vi "jiga.vi"() -> ()   [LabVIEW 2014]
uses:
  stateCtl.ctl
  <vilib>/Instr/_visa.llb/VISA Configure Serial Port (Instr).vi
panel:
  in  "Digital\nOutput 3":bool
  out "Led3":bool
  out "ASCII Read":string
  in  "Filter\nRead":bool
  out "Led0":bool
  out "ASCII Digital":string
  out "ASCII Analog 2":string
  out "ASCII Analog 1":string
  in  "AnalogOutput 2 \n      DutyCycle":dbl(slide) scale=0.0..100.0
  out "S7":dbl
  in  "AnalogOutput 1 \n      DutyCycle":dbl(slide) scale=0.0..100.0
  out "Led2":bool
  in  "Digital\nOutput 2":bool
  out "Led1":bool
  in  "Digital\nOutput 1":bool
  out "S6":dbl
  out "S5":dbl
  out "S4":dbl
  out "S3":dbl
  out "S2":dbl
  out "S1":dbl
  out "S0":dbl
  in  "Tab Control":T1(tab)
  out "Frequency":dbl(graph)
  out "Temperature 1":dbl(graph)
  out "Temperature 2":dbl(graph)
  out "Load Cell 1":dbl(graph)
  out "Load Cell 2":dbl(graph)
  out "Vibration":dbl(graph)
  out "Analog Output 1":dbl(graph)
  out "Analog Output 2":dbl(graph)
  out "exitLed":bool
  out "statusBar":string="     "
  in  "startButton":bool
  out "stopLed":bool
  out "startLed":bool
  in  "VISA Serial Port":refnum<visa-resource-name>
  in  "exitButton":bool
  in  "stopButton":bool
  out "FE":string
  out "FP":string
  out "isRunning":bool
  out "state":T2=enum."exit"
  # "`"
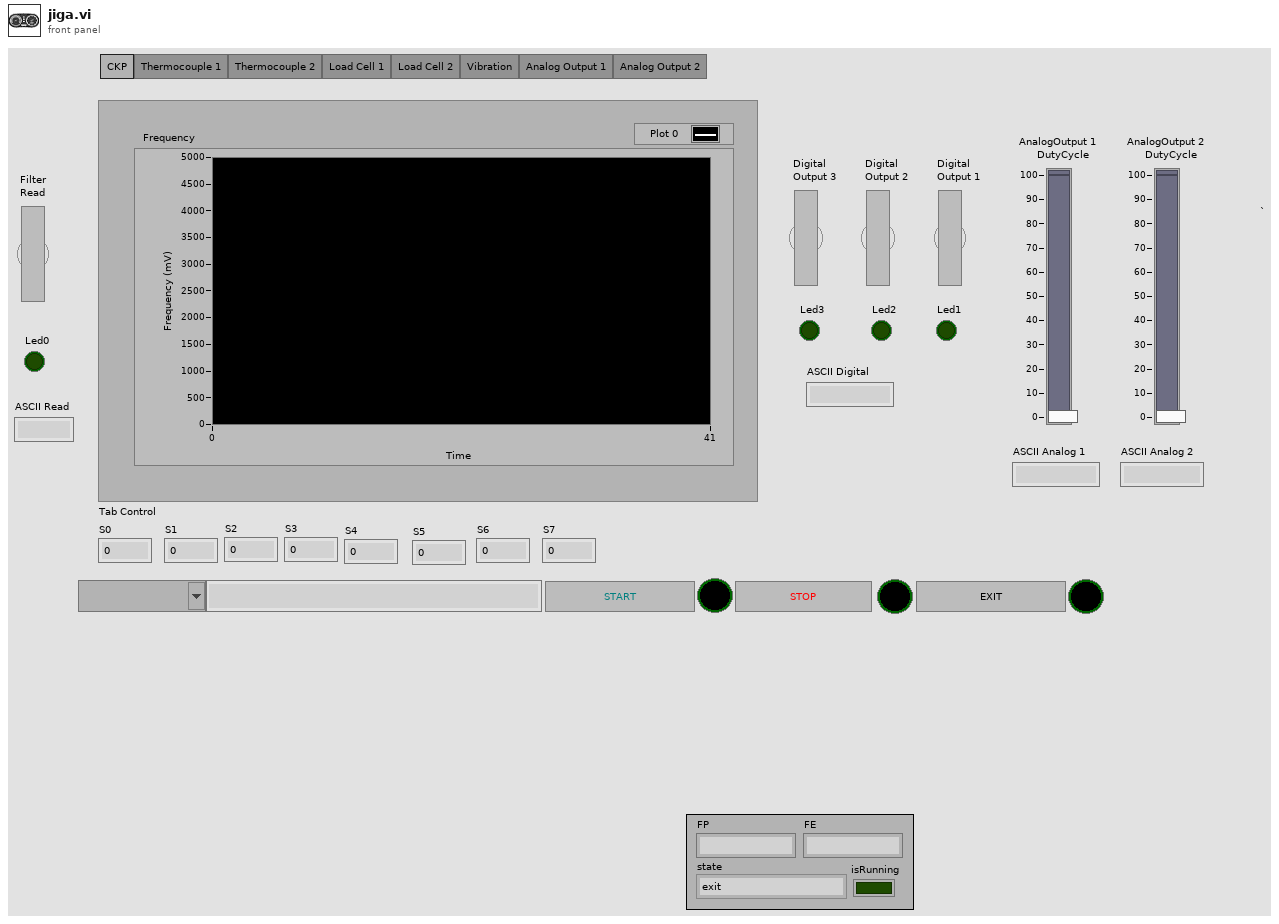
[diagram p1: front panel]
types:
  T1 = enum32{"CKP", "Thermocouple 1", "Thermocouple 2", "Load Cell 1", "Load Cell 2", "Vibration", "Analog Output 1", "Analog Output 2"}
  T2 = typedef "stateCtl.ctl" = enum16{"init", "ready", "running", "stopped", "exit"}
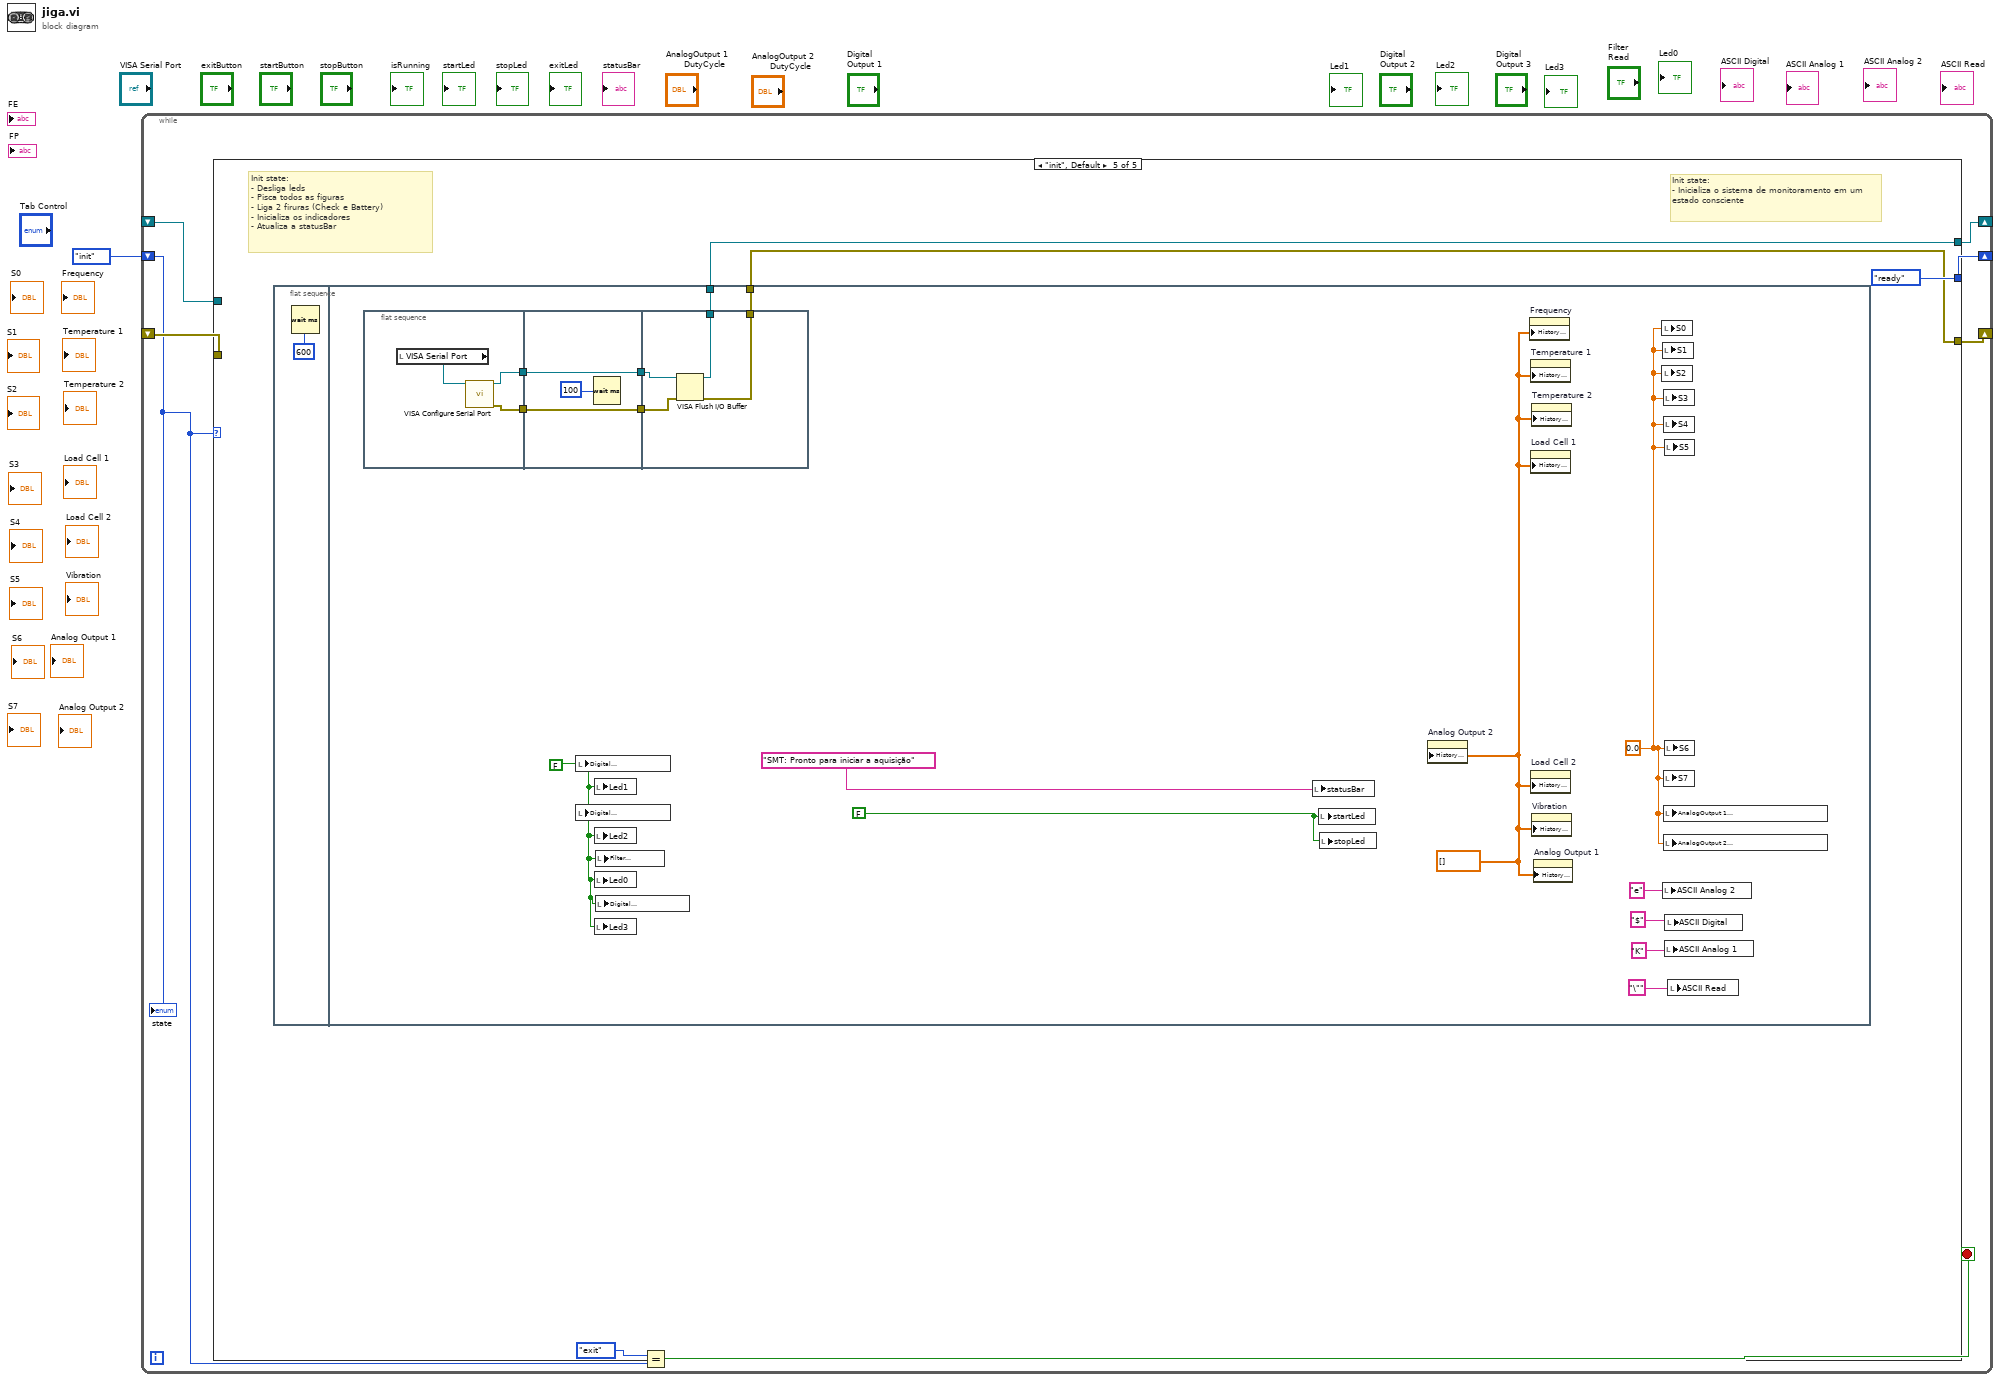
[diagram p0: block diagram]
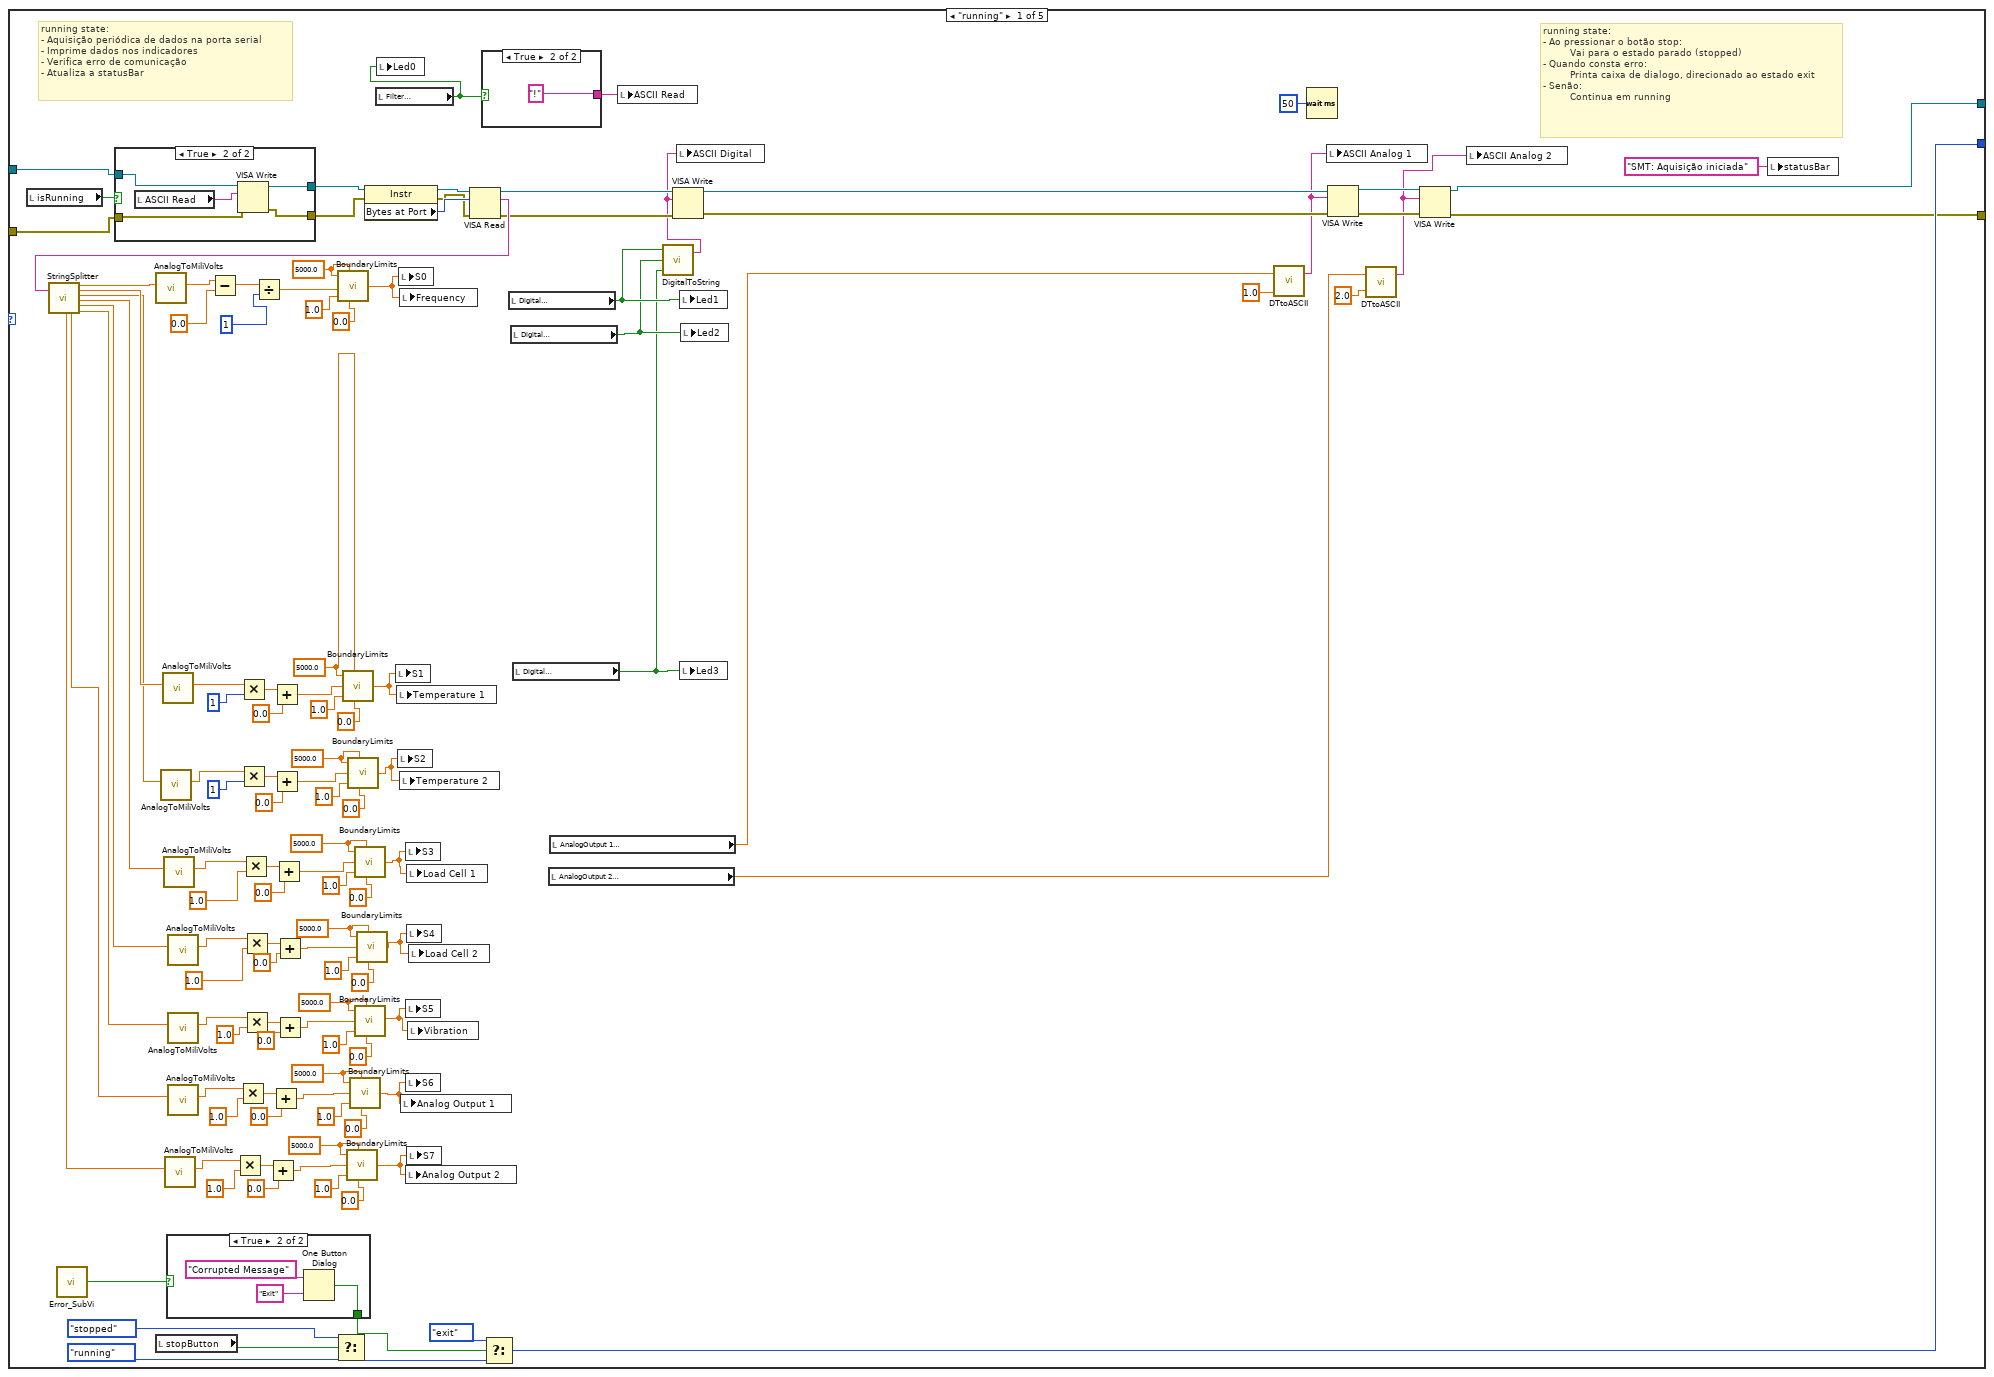
[diagram p2: hidden frame]
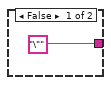
[diagram p3: hidden frame]
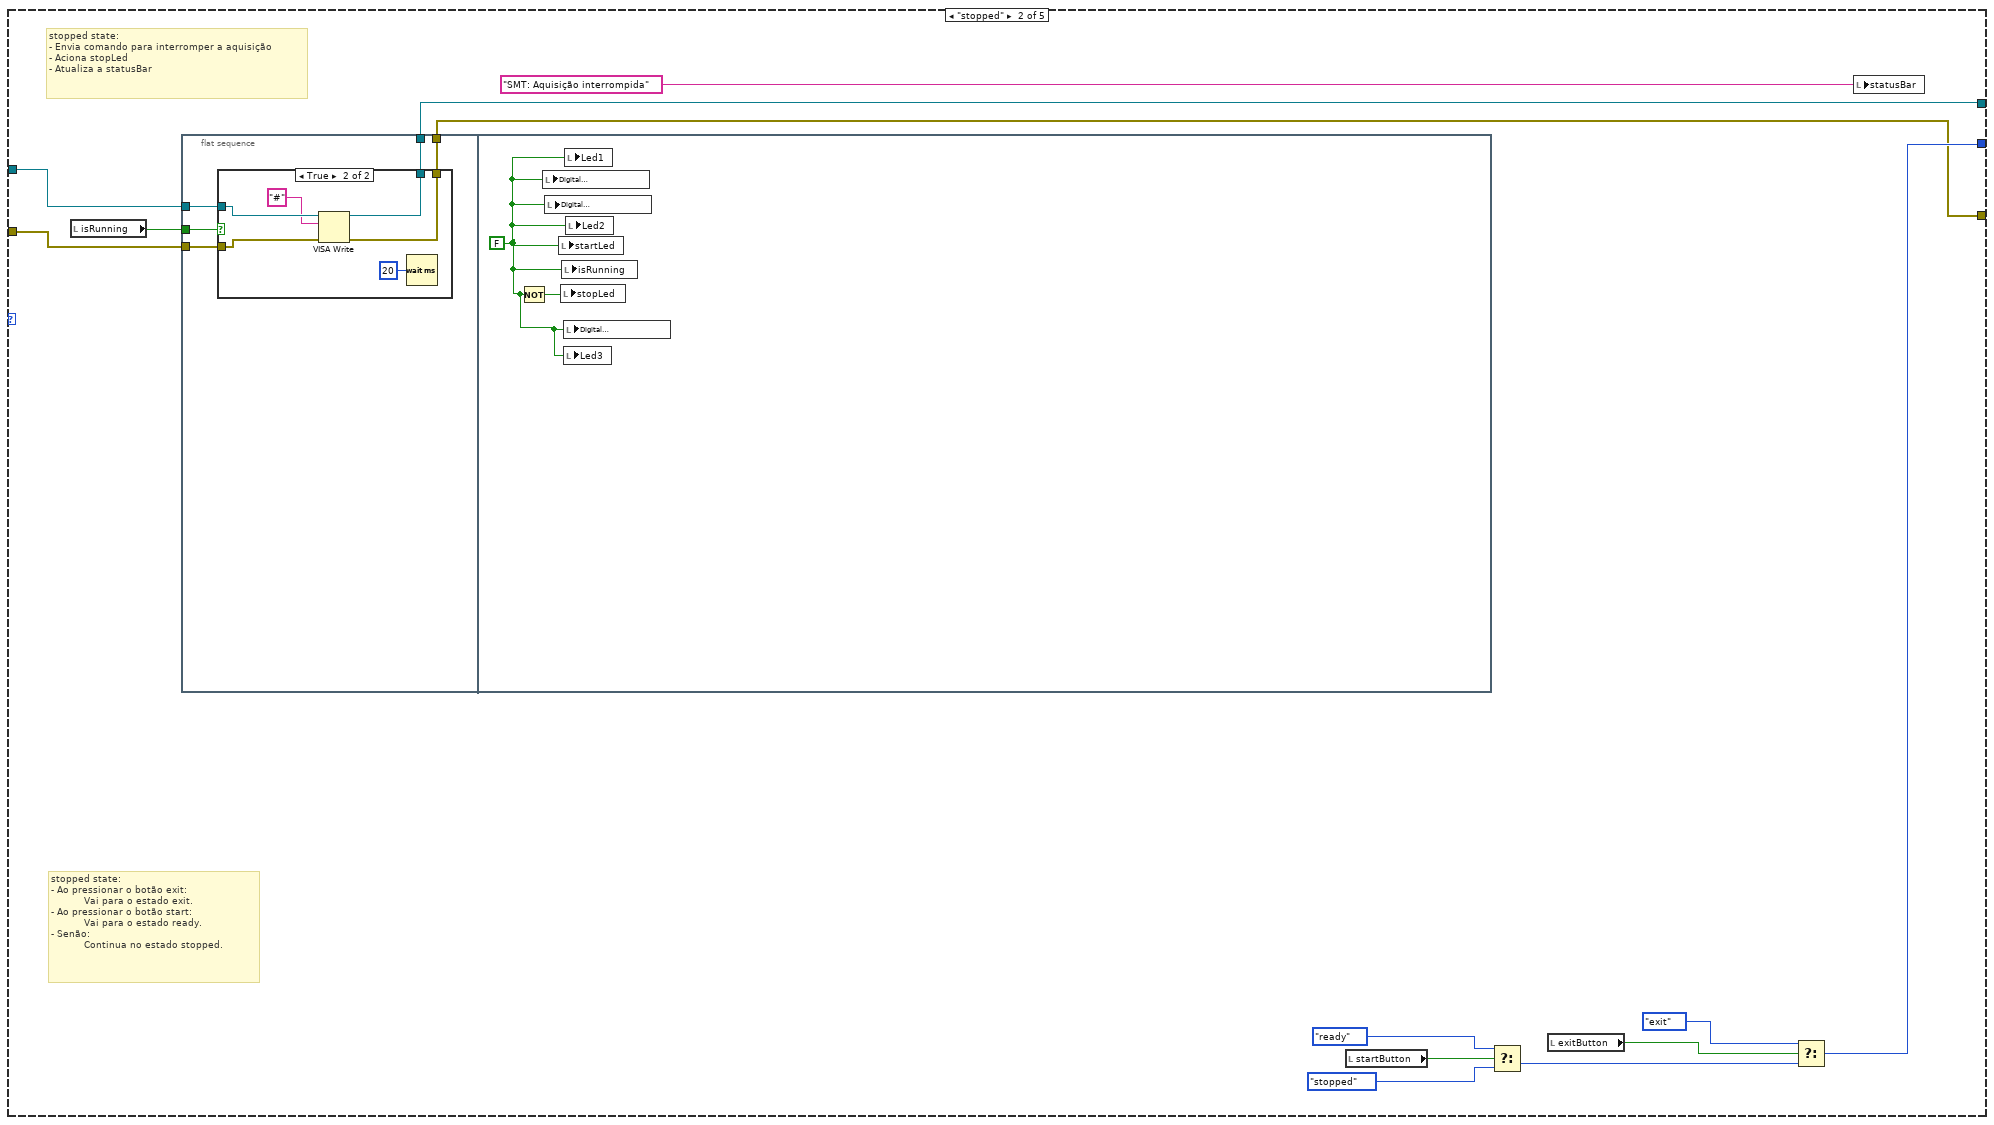
[diagram p6: hidden frame]
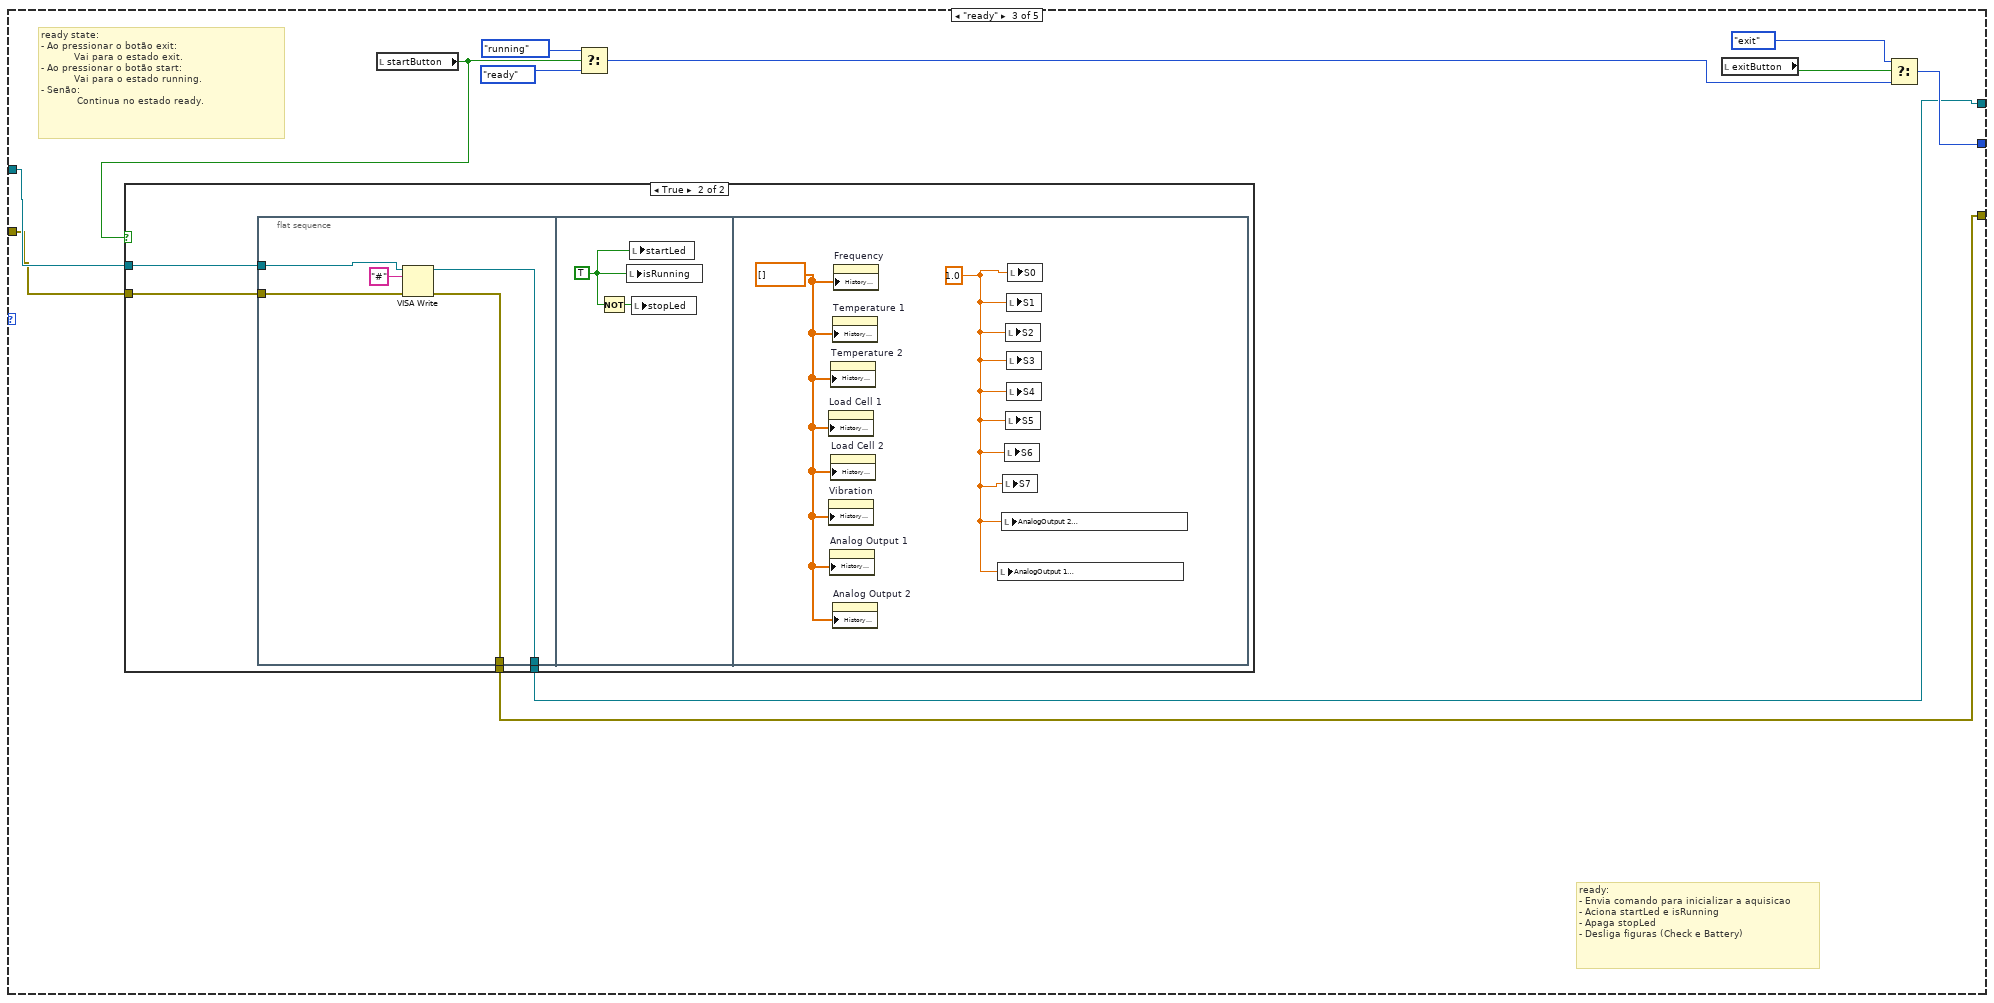
[diagram p8: hidden frame]
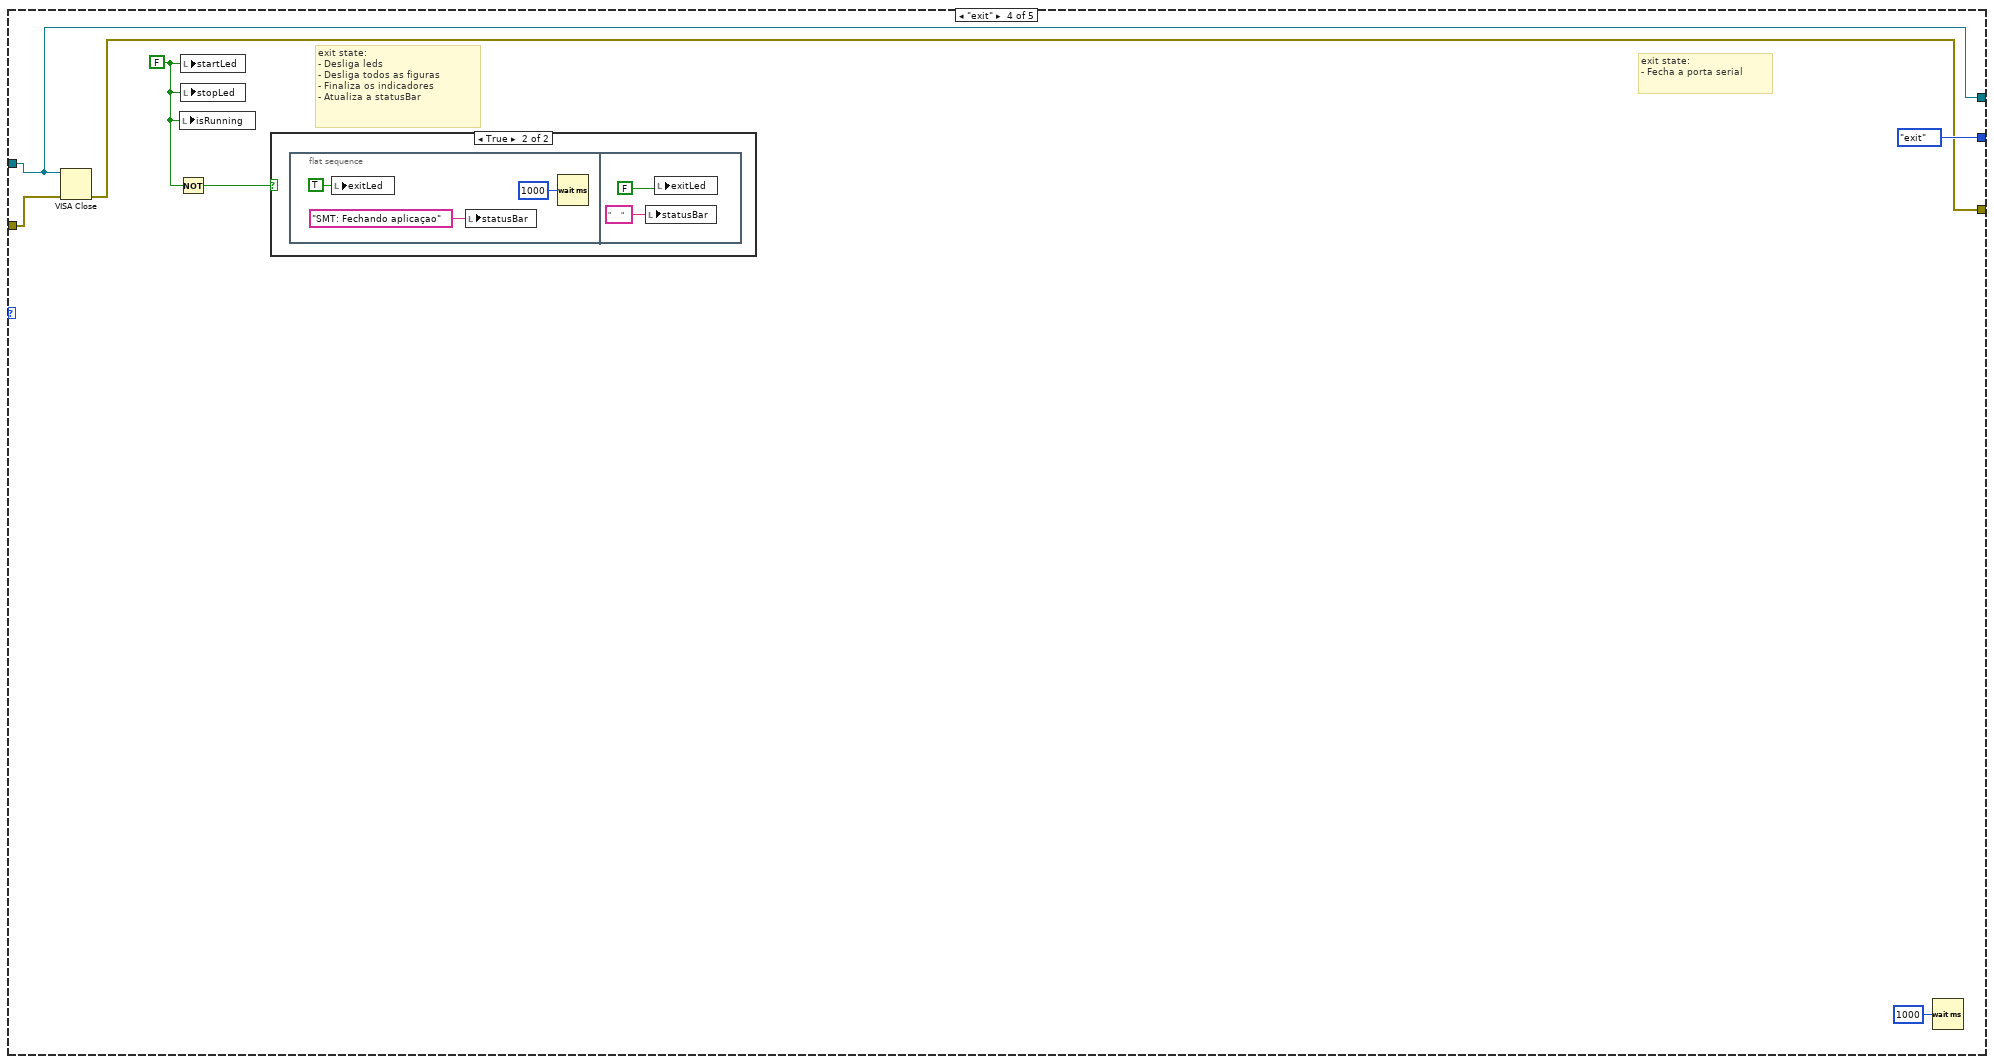
[diagram p10: hidden frame]
diagram:
  n1 = while {
    shift-right: [w3] -> _
    shift-left: _ -> [w8]
    shift-right: [w9] -> _
    shift-left: _ -> [w7]
    shift-right: [w4] -> _
    shift-left: stateCtl."init" ("state") -> [w5]
    stop <- w2 stop-if-true
    n2 = case shown="\"init\", Default" w5 {
      tunnel: [w27 w146 w171 w199 w209] -> w3
      tunnel: [w26 w147 w170 w200 w208] -> w9
      tunnel: [w122 w152 w175 stateCtl."exit" ("state") stateCtl."ready" ("state")] -> w4
      tunnel: w8 -> [w96 w150 w173 w199 _]
      tunnel: w7 -> [w95 w149 w172 w201 _]
      frame "running" {
        w40 = 5000.0
        w63 = 5000.0
        w66 = 5000.0
        w69 = 5000.0
        w74 = 5000.0
        w79 = 5000.0
        w84 = 5000.0
        w87 = 5000.0
        # "running state:\n- Ao pressionar o botão stop: \n         Vai para o estado parado (stopped)\n- Quando consta erro:\n         Printa caixa de dialogo, direcionado ao estado exit  \n- Senão:          \n         Continua em running"
        # "running state:\n- Aquisição periódica de dados na porta serial\n- Imprime dados nos indicadores\n- Verifica erro de comunicação\n- Atualiza a statusBar"
        n3 = local read "isRunning"() -> (w119:bool)
        n4 = call "Error_SubVi.vi"() -> ("error"=w118:bool)  [unwired: 11 in]
        n5 = case shown="True" w119 {
          tunnel: [w136 w138] -> w93
          tunnel: [w135 w139] -> w94
          tunnel: w95 -> [w136 w141]
          tunnel: w96 -> [w135 w140]
          frame False {
          }
          frame True {
            n6 = local read "ASCII Read"() -> (w137:string)
            n7 = VISA Write(VISA resource name=w140, write buffer=w137, error in (no error)=w141) -> (VISA resource name out=w139:refnum<visa-resource-name>, error out=w138:errorcluster)  [unwired: 1 out]
          }
        }
        n8 = local read "stopButton"() -> (w126:bool)
        n9 = case shown="True" w118 {
          selector: w118 -> [w131 _]
          tunnel: [w131 w132] -> w120
          frame False {
          }
          frame True {
            n10 = One Button Dialog(message="Corrupted Message", button name ("OK")="Exit") -> (true=w132:bool)
          }
        }
        n11 = Select(t=stateCtl."stopped" ("state"), s=w126, f=stateCtl."running" ("state")) -> (s? t:f=w121:T2)
        n12 = property class="Instr"(reference=w94, error in=w93) -> (reference out=w90:refnum<visa-resource-name>, error out=w91:errorcluster, "Bytes at Port"=w92:u32)
        n13 = local read "Filter\nRead"() -> (w20:bool)
        n14 = local write "Led0"(w20) -> ()
        n15 = VISA Read(VISA resource name=w90, byte count=w92, error in (no error)=w91) -> (VISA resource name out=w44:refnum<visa-resource-name>, read buffer=w89:string, error out=w43:errorcluster)  [unwired: 1 out]
        n16 = call "StringSplitter.vi"("Input String"=w89) -> ("S7"=w33:dbl, "S6"=w97:dbl, "S0"=w103:dbl, "S1"=w102:dbl, "S2"=w101:dbl, "S3"=w100:dbl, "S4"=w99:dbl, "S5"=w98:dbl)  [unwired: 11 in]
        n17 = call "AnalogToMiliVolts.vi"("Input"=w103) -> ("Output"=w18:dbl)  [unwired: 10 in]
        n18 = call "AnalogToMiliVolts.vi"("Input"=w101) -> ("Output"=w105:dbl)  [unwired: 10 in]
        n19 = call "AnalogToMiliVolts.vi"("Input"=w102) -> ("Output"=w104:dbl)  [unwired: 10 in]
        n20 = call "AnalogToMiliVolts.vi"("Input"=w100) -> ("Output"=w106:dbl)  [unwired: 10 in]
        n21 = call "AnalogToMiliVolts.vi"("Input"=w33) -> ("Output"=w41:dbl)  [unwired: 10 in]
        n22 = call "AnalogToMiliVolts.vi"("Input"=w99) -> ("Output"=w107:dbl)  [unwired: 10 in]
        n23 = call "AnalogToMiliVolts.vi"("Input"=w98) -> ("Output"=w108:dbl)  [unwired: 10 in]
        n24 = call "AnalogToMiliVolts.vi"("Input"=w97) -> ("Output"=w109:dbl)  [unwired: 10 in]
        n25 = Subtract(x=w18, y=0.0) -> (x-y=w15:dbl)
        n26 = Multiply(x=w41, y=1.0) -> (x*y=w42:dbl)
        n27 = Multiply(x=w109, y=1.0) -> (x*y=w110:dbl)
        n28 = Multiply(x=w104, y=1) -> (x*y=w116:dbl)
        n29 = Multiply(x=w105, y=1) -> (x*y=w114:dbl)
        n30 = Multiply(x=w106, y=1.0) -> (x*y=w113:dbl)
        n31 = Multiply(x=w107, y=1.0) -> (x*y=w112:dbl)
        n32 = Multiply(x=w108, y=1.0) -> (x*y=w111:dbl)
        n33 = Divide(x=w15, y=1) -> (x/y=w14:dbl)
        n34 = Add(x=w42, y=0.0) -> (x+y=w36:dbl)
        n35 = Add(x=w110, y=0.0) -> (x+y=w54:dbl)
        n36 = Add(x=w116, y=0.0) -> (x+y=w81:dbl)
        n37 = Add(x=w114, y=0.0) -> (x+y=w76:dbl)
        n38 = Add(x=w113, y=0.0) -> (x+y=w70:dbl)
        n39 = Add(x=w112, y=0.0) -> (x+y=w52:dbl)
        n40 = Add(x=w111, y=0.0) -> (x+y=w53:dbl)
        n41 = call "BoundaryLimits.vi"("UpperLimit"=w87, "UpperValue"=w87, "Input"=w14, "LowerLimit"=1.0, "LowerValue"=0.0) -> ("Output"=w88:dbl)
        n42 = call "BoundaryLimits.vi"("UpperLimit"=w84, "UpperValue"=w84, "Input"=w81, "LowerLimit"=1.0, "LowerValue"=0.0) -> ("Output"=w80:dbl)
        n43 = call "BoundaryLimits.vi"("UpperLimit"=w40, "UpperValue"=w40, "Input"=w36, "LowerLimit"=1.0, "LowerValue"=0.0) -> ("Output"=w34:dbl)
        n44 = call "BoundaryLimits.vi"("UpperLimit"=w79, "UpperValue"=w79, "Input"=w76, "LowerLimit"=1.0, "LowerValue"=0.0) -> ("Output"=w75:dbl)
        n45 = call "BoundaryLimits.vi"("UpperLimit"=w63, "UpperValue"=w63, "Input"=w54, "LowerLimit"=1.0, "LowerValue"=0.0) -> ("Output"=w49:dbl)
        n46 = call "BoundaryLimits.vi"("UpperLimit"=w74, "UpperValue"=w74, "Input"=w70, "LowerLimit"=1.0, "LowerValue"=0.0) -> ("Output"=w71:dbl)
        n47 = call "BoundaryLimits.vi"("UpperLimit"=w66, "UpperValue"=w66, "Input"=w53, "LowerLimit"=1.0, "LowerValue"=0.0) -> ("Output"=w50:dbl)
        n48 = call "BoundaryLimits.vi"("UpperLimit"=w69, "UpperValue"=w69, "Input"=w52, "LowerLimit"=1.0, "LowerValue"=0.0) -> ("Output"=w51:dbl)
        n49 = local write "S1"(w80) -> ()
        n50 = local write "Temperature 1"(w80) -> ()
        n51 = local write "S2"(w75) -> ()
        n52 = local write "S0"(w88) -> ()
        n53 = local write "Frequency"(w88) -> ()
        n54 = local write "Temperature 2"(w75) -> ()
        n55 = local write "Analog Output 1"(w49) -> ()
        n56 = local write "S3"(w71) -> ()
        n57 = local write "S5"(w50) -> ()
        n58 = local write "S6"(w49) -> ()
        n59 = local write "Analog Output 2"(w34) -> ()
        n60 = local write "Load Cell 1"(w71) -> ()
        n61 = local write "S4"(w51) -> ()
        n62 = local write "S7"(w34) -> ()
        n63 = local write "Vibration"(w50) -> ()
        n64 = local write "Load Cell 2"(w51) -> ()
        n65 = case shown="True" w20 {
          tunnel: ["\"" ("write buffer") "!" ("write buffer")] -> w19
          frame False {
          }
          frame True {
          }
        }
        n66 = Select(t=stateCtl."exit" ("state"), s=w120, f=w121) -> (s? t:f=w122:T2)
        n67 = local read "Digital\nOutput 1"() -> (w12:bool)
        n68 = local read "Digital\nOutput 2"() -> (w11:bool)
        n69 = local read "Digital\nOutput 3"() -> (w10:bool)
        n70 = local read "AnalogOutput 2 \n      DutyCycle"() -> (w25:dbl)
        n71 = local read "AnalogOutput 1 \n      DutyCycle"() -> (w32:dbl)
        n72 = local write "ASCII Read"(w19) -> ()
        n73 = call "DigitalToString.vi"("D3"=w10, "D2"=w11, "D1"=w12) -> ("String"=w13:string)  [unwired: 1 out]
        n74 = VISA Write(VISA resource name=w44, write buffer=w13, error in (no error)=w43) -> (VISA resource name out=w30:refnum<visa-resource-name>, error out=w31:errorcluster)  [unwired: 1 out]
        n75 = local write "ASCII Digital"(w13) -> ()
        n76 = local write "Led1"(w12) -> ()
        n77 = local write "Led3"(w10) -> ()
        n78 = local write "Led2"(w11) -> ()
        n79 = call "DTtoASCII.vi"("Channel"=1.0, "Slide"=w32) -> ("ASCII"=w21:string)  [unwired: 1 out]
        n80 = Wait (ms)(milliseconds to wait=u32 50) -> ()  [unwired: 1 out]
        n81 = local write "ASCII Analog 1"(w21) -> ()
        n82 = VISA Write(VISA resource name=w30, write buffer=w21, error in (no error)=w31) -> (VISA resource name out=w28:refnum<visa-resource-name>, error out=w29:errorcluster)  [unwired: 1 out]
        n83 = call "DTtoASCII.vi"("Channel"=2.0, "Slide"=w25) -> ("ASCII"=w22:string)  [unwired: 1 out]
        n84 = VISA Write(VISA resource name=w28, write buffer=w22, error in (no error)=w29) -> (VISA resource name out=w27:refnum<visa-resource-name>, error out=w26:errorcluster)  [unwired: 1 out]
        n85 = local write "ASCII Analog 2"(w22) -> ()
        n86 = local write "statusBar"("SMT: Aquisição iniciada" ("statusBar")) -> ()
      }
      frame "stopped" {
        # "stopped state:\n- Ao pressionar o botão exit: \n           Vai para o estado exit.\n- Ao pressionar o botão start:\n           Vai para o estado ready.\n- Senão:\n           Continua no estado stopped."
        # "stopped state:\n- Envia comando para interromper a aquisição\n- Aciona stopLed\n- Atualiza a statusBar"
        n87 = local read "isRunning"() -> (w148:bool)
        n88 = flat-sequence {
          tunnel: w150 -> [w159]
          tunnel: w149 -> [w158]
          tunnel: w148 -> [w157]
          tunnel: [w156] -> w147
          tunnel: [w155] -> w146
          frame #0 {
            n89 = case shown="True" w157 {
              tunnel: w159 -> [w161 w167]
              tunnel: w158 -> [w160 w166]
              tunnel: [w160 w162] -> w156
              tunnel: [w161 w164] -> w155
              frame False {
              }
              frame True {
                n90 = VISA Write(VISA resource name=w167, write buffer="#", error in (no error)=w166) -> (VISA resource name out=w164:refnum<visa-resource-name>, error out=w162:errorcluster)  [unwired: 1 out]
                n91 = Wait (ms)(milliseconds to wait=u32 20) -> ()  [unwired: 1 out]
              }
            }
          }
          frame #1 {
            w168 = FALSE ("Boolean")
            n92 = Not(x=w168) -> (.not. x?=w169:bool)
            n93 = local write "Digital\nOutput 1"(w168) -> ()
            n94 = local write "Digital\nOutput 2"(w168) -> ()
            n95 = local write "startLed"(w168) -> ()
            n96 = local write "stopLed"(w169) -> ()
            n97 = local write "isRunning"(w168) -> ()
            n98 = local write "Digital\nOutput 3"(w168) -> ()
            n99 = local write "Led3"(w168) -> ()
            n100 = local write "Led1"(w168) -> ()
            n101 = local write "Led2"(w168) -> ()
          }
        }
        n102 = local read "startButton"() -> (w145:bool)
        n103 = Select(t=stateCtl."ready" ("state"), s=w145, f=stateCtl."stopped" ("state")) -> (s? t:f=w153:T2)
        n104 = local read "exitButton"() -> (w144:bool)
        n105 = Select(t=stateCtl."exit" ("state"), s=w144, f=w153) -> (s? t:f=w152:T2)
        n106 = local write "statusBar"("SMT: Aquisição interrompida" ("statusBar")) -> ()
      }
      frame "ready" {
        # "ready state:\n- Ao pressionar o botão exit: \n           Vai para o estado exit.\n- Ao pressionar o botão start:\n           Vai para o estado running.\n- Senão:\n            Continua no estado ready."
        # "ready:\n- Envia comando para inicializar a aquisicao\n- Aciona startLed e isRunning\n- Apaga stopLed\n- Desliga figuras (Check e Battery)"
        n107 = local read "startButton"() -> (w174:bool)
        n108 = case shown="True" w174 {
          tunnel: w173 -> [w182 w186]
          tunnel: w172 -> [w181 w185]
          tunnel: [w182 w184] -> w171
          tunnel: [w181 w183] -> w170
          frame False {
          }
          frame True {
            n109 = flat-sequence {
              tunnel: w186 -> [w190]
              tunnel: w185 -> [w189]
              tunnel: [w188] -> w184
              tunnel: [w187] -> w183
              frame #0 {
                n110 = VISA Write(VISA resource name=w190, write buffer="#", error in (no error)=w189) -> (VISA resource name out=w188:refnum<visa-resource-name>, error out=w187:errorcluster)  [unwired: 1 out]
              }
              frame #1 {
                w193 = TRUE ("Boolean")
                n111 = Not(x=w193) -> (.not. x?=w192:bool)
                n112 = local write "isRunning"(w193) -> ()
                n113 = local write "startLed"(w193) -> ()
                n114 = local write "stopLed"(w192) -> ()
              }
              frame #2 {
                w194 = 1.0
                w195 = dbl[] [] ("History Data")
                n115 = property on="Load Cell 1" class="WFChart (strict)"("History Data"=w195) -> ()  [unwired: 2 in, 2 out]
                n116 = property on="Vibration" class="WFChart (strict)"("History Data"=w195) -> ()  [unwired: 2 in, 2 out]
                n117 = property on="Analog Output 1" class="WFChart (strict)"("History Data"=w195) -> ()  [unwired: 2 in, 2 out]
                n118 = property on="Temperature 2" class="WFChart (strict)"("History Data"=w195) -> ()  [unwired: 2 in, 2 out]
                n119 = property on="Load Cell 2" class="WFChart (strict)"("History Data"=w195) -> ()  [unwired: 2 in, 2 out]
                n120 = property on="Temperature 1" class="WFChart (strict)"("History Data"=w195) -> ()  [unwired: 2 in, 2 out]
                n121 = property on="Analog Output 2" class="WFChart (strict)"("History Data"=w195) -> ()  [unwired: 2 in, 2 out]
                n122 = property on="Frequency" class="WFChart (strict)"("History Data"=w195) -> ()  [unwired: 2 in, 2 out]
                n123 = local write "AnalogOutput 1 \n      DutyCycle"(w194) -> ()
                n124 = local write "AnalogOutput 2 \n      DutyCycle"(w194) -> ()
                n125 = local write "S7"(w194) -> ()
                n126 = local write "S6"(w194) -> ()
                n127 = local write "S2"(w194) -> ()
                n128 = local write "S5"(w194) -> ()
                n129 = local write "S1"(w194) -> ()
                n130 = local write "S3"(w194) -> ()
                n131 = local write "S4"(w194) -> ()
                n132 = local write "S0"(w194) -> ()
              }
            }
          }
        }
        n133 = Select(t=stateCtl."running" ("state"), s=w174, f=stateCtl."ready" ("state")) -> (s? t:f=w176:T2)
        n134 = local read "exitButton"() -> (w178:bool)
        n135 = Select(t=stateCtl."exit" ("state"), s=w178, f=w176) -> (s? t:f=w175:T2)
      }
      frame "exit" {
        w197 = FALSE ("startLed")
        # "exit state:\n- Desliga leds\n- Desliga todos as figuras\n- Finaliza os indicadores\n- Atualiza a statusBar"
        # "exit state:\n- Fecha a porta serial"
        n136 = VISA Close(VISA resource name=w199, error in (no error)=w201) -> (error out=w200:errorcluster)
        n137 = Not(x=w197) -> (.not. x?=w198:bool)
        n138 = local write "isRunning"(w197) -> ()
        n139 = local write "startLed"(w197) -> ()
        n140 = local write "stopLed"(w197) -> ()
        n141 = case shown="True" w198 {
          frame False {
          }
          frame True {
            n142 = flat-sequence {
              frame #0 {
                n143 = local write "exitLed"(TRUE ("exitLed")) -> ()
                n144 = local write "statusBar"("SMT: Fechando aplicaçao" ("statusBar")) -> ()
                n145 = Wait (ms)(milliseconds to wait=u32 1000) -> ()  [unwired: 1 out]
              }
              frame #1 {
                n146 = local write "statusBar"("     " ("statusBar")) -> ()
                n147 = local write "exitLed"(FALSE ("exitLed")) -> ()
              }
            }
          }
        }
        n148 = Wait (ms)(milliseconds to wait=u32 1000) -> ()  [unwired: 1 out]
      }
      frame "init", Default {
        # "Init state:\n- Inicializa o sistema de monitoramento em um estado consciente"
        # "Init state:\n- Desliga leds\n- Pisca todos as figuras\n- Liga 2 firuras (Check e Battery)\n- Inicializa os indicadores\n- Atualiza a statusBar"
        n149 = flat-sequence {
          tunnel: [w213] -> w209
          tunnel: [w212] -> w208
          frame #0 {
            n150 = Wait (ms)(milliseconds to wait=u32 600) -> ()  [unwired: 1 out]
          }
          frame #1 {
            w224 = dbl[] [] ("History Data")
            w223 = 0.0
            w218 = FALSE
            w226 = FALSE
            n151 = flat-sequence {
              tunnel: [w228] -> w216
              tunnel: [w227] -> w215
              tunnel: [w231] -> w217
              tunnel: w216 -> [w231]
              tunnel: w215 -> [w230]
              tunnel: [w230] -> w214
              tunnel: w217 -> [w236]
              tunnel: w214 -> [w235]
              tunnel: [w234] -> w213
              tunnel: [w233] -> w212
              frame #0 {
                n152 = local read "VISA Serial Port"() -> (w229:refnum<visa-resource-name>)
                n153 = call-poly "VISA Configure Serial Port"("VISA resource name"=w229) -> ("VISA resource name out"=w228:refnum<visa-resource-name>, "error out"=w227:errorcluster)  [unwired: 13 in]
              }
              frame #1 {
                n154 = Wait (ms)(milliseconds to wait=u32 100) -> ()  [unwired: 1 out]
              }
              frame #2 {
                n155 = VISA Flush I/O Buffer(VISA resource name=w236, error in (no error)=w235) -> (VISA resource name out=w234:refnum<visa-resource-name>, error out=w233:errorcluster)  [unwired: 1 in]
              }
            }
            n156 = local write "Digital\nOutput 1"(w218) -> ()
            n157 = local write "Digital\nOutput 2"(w218) -> ()
            n158 = local write "Led1"(w218) -> ()
            n159 = local write "Led2"(w218) -> ()
            n160 = local write "Led0"(w218) -> ()
            n161 = local write "Led3"(w218) -> ()
            n162 = local write "Filter\nRead"(w218) -> ()
            n163 = local write "Digital\nOutput 3"(w218) -> ()
            n164 = local write "statusBar"("SMT: Pronto para iniciar a aquisição" ("statusBar")) -> ()
            n165 = local write "startLed"(w226) -> ()
            n166 = local write "stopLed"(w226) -> ()
            n167 = property on="Analog Output 2" class="WFChart (strict)"("History Data"=w224) -> ()  [unwired: 2 in, 2 out]
            n168 = property on="Frequency" class="WFChart (strict)"("History Data"=w224) -> ()  [unwired: 2 in, 2 out]
            n169 = property on="Temperature 1" class="WFChart (strict)"("History Data"=w224) -> ()  [unwired: 2 in, 2 out]
            n170 = property on="Load Cell 1" class="WFChart (strict)"("History Data"=w224) -> ()  [unwired: 2 in, 2 out]
            n171 = property on="Load Cell 2" class="WFChart (strict)"("History Data"=w224) -> ()  [unwired: 2 in, 2 out]
            n172 = property on="Temperature 2" class="WFChart (strict)"("History Data"=w224) -> ()  [unwired: 2 in, 2 out]
            n173 = property on="Vibration" class="WFChart (strict)"("History Data"=w224) -> ()  [unwired: 2 in, 2 out]
            n174 = property on="Analog Output 1" class="WFChart (strict)"("History Data"=w224) -> ()  [unwired: 2 in, 2 out]
            n175 = local write "S0"(w223) -> ()
            n176 = local write "S2"(w223) -> ()
            n177 = local write "S1"(w223) -> ()
            n178 = local write "ASCII Analog 2"("e") -> ()
            n179 = local write "S3"(w223) -> ()
            n180 = local write "S4"(w223) -> ()
            n181 = local write "S7"(w223) -> ()
            n182 = local write "AnalogOutput 1 \n      DutyCycle"(w223) -> ()
            n183 = local write "AnalogOutput 2 \n      DutyCycle"(w223) -> ()
            n184 = local write "S5"(w223) -> ()
            n185 = local write "S6"(w223) -> ()
            n186 = local write "ASCII Analog 1"("K") -> ()
            n187 = local write "ASCII Digital"("$") -> ()
            n188 = local write "ASCII Read"("\"") -> ()
          }
        }
      }
    }
    n189 = Equal?(x=stateCtl."exit" ("state"), y=w5) -> (x = y?=w2:bool)
    "state" <- w5
  }
